vi "Calculator.vi"() -> ()   [LabVIEW 2014]
panel:
  out "Numeric 3":dbl
  in  "Numeric 2":dbl
  in  "Numeric":dbl
  out "Multiply":bool
  out "Add":bool
  out "Subtract":bool
  in  "Slide":i8(slide) scale=0.0..2.0
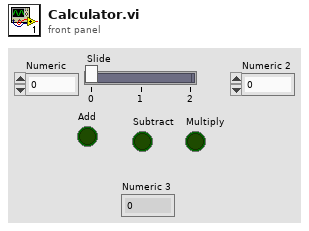
[diagram p1: front panel]
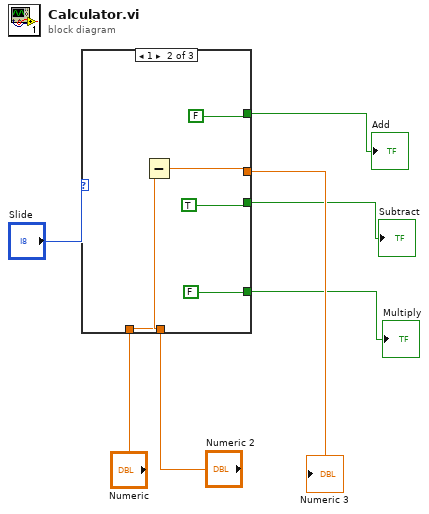
[diagram p0: block diagram]
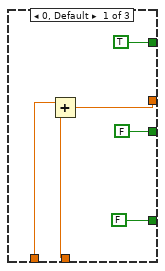
[diagram p2: hidden frame]
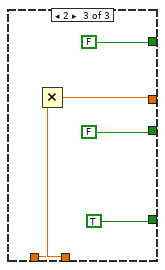
[diagram p3: hidden frame]
diagram:
  n1 = case shown="1" "Slide" {
    tunnel: "Numeric 2" -> [w12 w18 w24]
    tunnel: "Numeric" -> [w11 w17 w23]
    tunnel: [w13 w19 w25] -> w5
    tunnel: [FALSE FALSE TRUE] -> w3
    tunnel: [FALSE TRUE FALSE] -> w2
    tunnel: [TRUE FALSE FALSE] -> w1
    frame 0, Default {
      n2 = Add(x=w11, y=w12) -> (x+y=w13:dbl)
    }
    frame 1 {
      n3 = Subtract(x=w17, y=w18) -> (x-y=w19:dbl)
    }
    frame 2 {
      n4 = Multiply(x=w23, y=w24) -> (x*y=w25:dbl)
    }
  }
  "Subtract" <- w2
  "Add" <- w1
  "Multiply" <- w3
  "Numeric 3" <- w5
